vi "GetTabDecorations.vi"(7 "decorations":i32[](array[numeric]), 9 "PythonConverter_GUI in":refnum<class "PythonConverter_GUI.lvclass">) -> (3 "PythonConverter_GUI out":refnum<class "PythonConverter_GUI.lvclass">, 5 "create_decorations":string)   [LabVIEW 2014, in "Raspberry Pi Compatible Compiler for LabVIEW.lvlib" / "PythonConverter_GUI.lvclass"]
uses:
  PythonConverter_GUI.lvclass
  Parsing/ClassTypeTD.ctl
  PythonConverter_GUI.lvclass/PythonConverter_GUI.ctl
  Parsing/Python Functions.lvlib
  VI Interpreter/Classes/VI Interpreter/VI Interpreter.lvclass
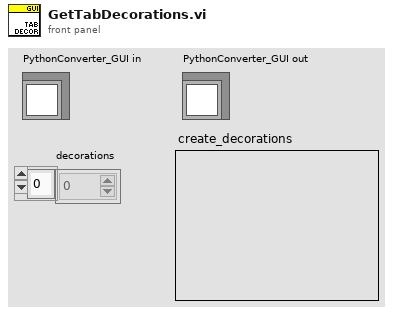
[diagram p1: front panel]
types:
  T1 = typedef "Raspberry Pi Compatible Compiler for LabVIEW.lvlib/Python Functions.lvlib/ClassTypeTD.ctl" = enum16{"class", "function"}
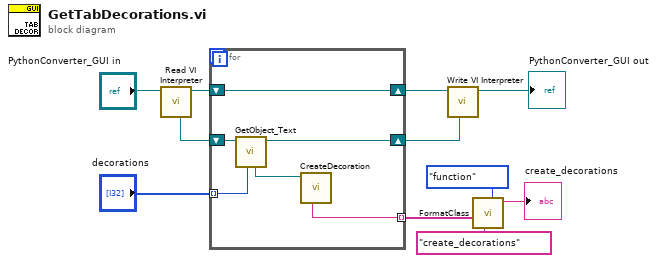
[diagram p0: block diagram]
diagram:
  n1 = call "Read VI Interpreter.vi"("PythonConverter_GUI in"="PythonConverter_GUI in") -> ("PythonConverter_GUI out"=w3:refnum<class "PythonConverter_GUI.lvclass">, "VI Interpreter"=w2:refnum<class "VI Interpreter.lvclass">)  [unwired: 7 in]
  n2 = for {
    tunnel: "decorations" -> [w16] mode=indexing
    shift-right: [w12] -> w6
    shift-left: w2 -> [w17]
    shift-right: [w15] -> w7
    shift-left: w3 -> [w15]
    tunnel: [w13] -> w1 mode=indexing
    n3 = call "GetObject_Text.vi"("UID"=w16, "VI Interpreter in"=w17) -> ("VI Interpreter out"=w12:refnum<class "VI Interpreter.lvclass">, "Text"=w14:refnum<class "Text.lvclass">)  [unwired: 4 in, 2 out]
    n4 = call "CreateDecoration.vi"("Decoration in"=w14) -> ("decoration"=w13:string)  [unwired: 7 in, 3 out]
  }
  n5 = call "Write VI Interpreter.vi"("VI Interpreter"=w6, "PythonConverter_GUI in"=w7) -> ("PythonConverter_GUI out"=→"PythonConverter_GUI out":refnum<class "PythonConverter_GUI.lvclass">)  [unwired: 7 in]
  n6 = call "FormatClass.vi"("type"=ClassTypeTD."function", "name"="create_decorations", "body"=w1) -> ("python"=→"create_decorations":string)  [unwired: 8 in]
